vi "Get Codec - copy.vi"(8 "error in (no error)":errorcluster, 10 "Codec In":string, 11 "Absolute Path":path) -> (0 "error out":errorcluster, 3 "Codec Out":string)   [LabVIEW 2020]
doc: "Determines supported audio codec name based on file extension or wired in codec string."
uses:
  <vilib>/Utility/error.llb/Error Cluster From Error Code.vi
  <vilib>/ErrorRing/Error Ring.xnode
  <vilib>/Dataflow_G/G-Audio/G-Audio.lvlib
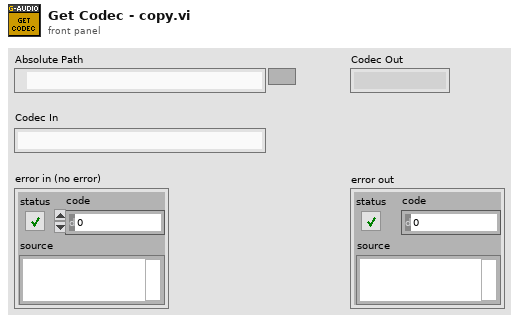
[diagram p1: front panel]
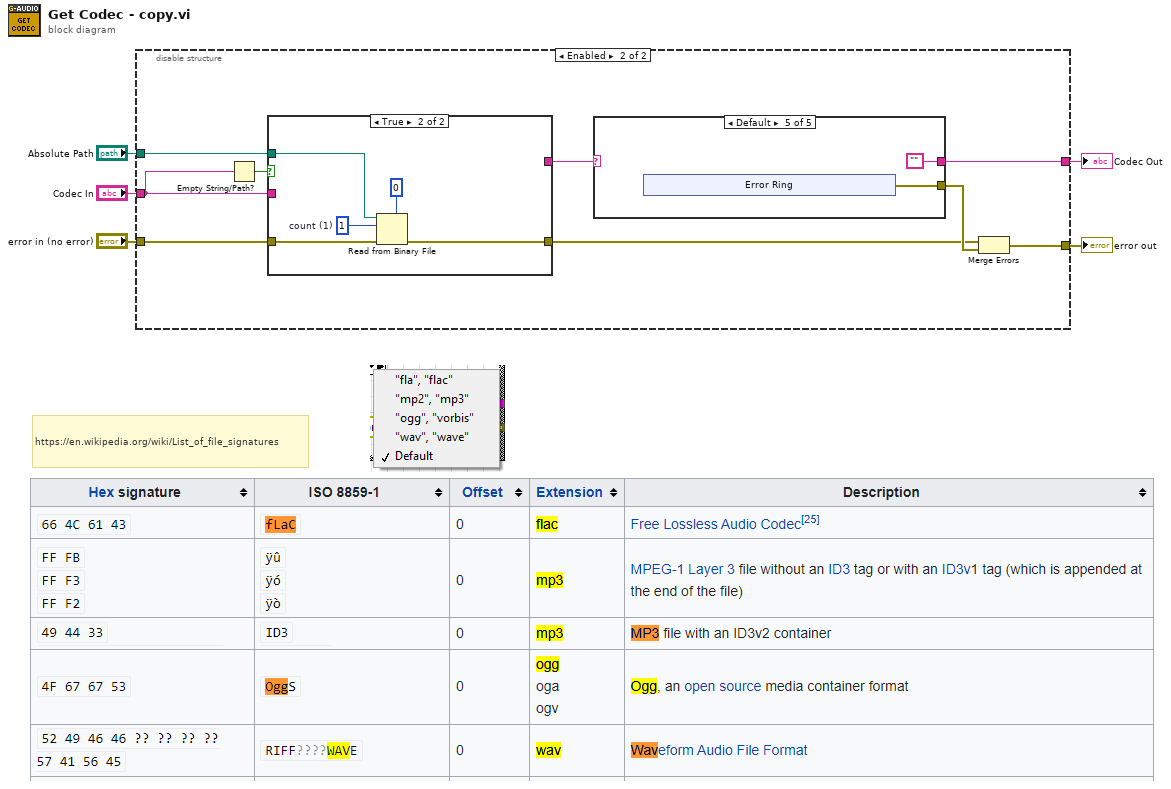
[diagram p0: block diagram]
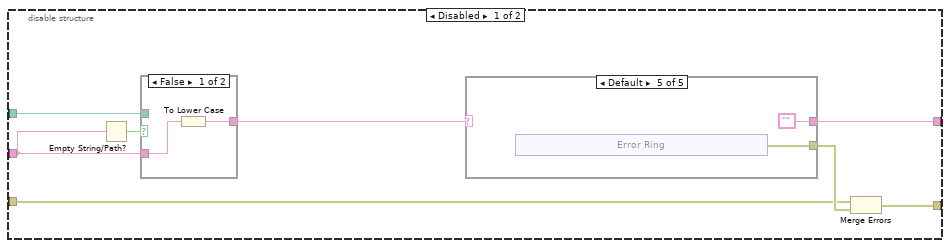
[diagram p2: hidden frame]
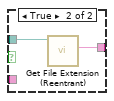
[diagram p3: hidden frame]
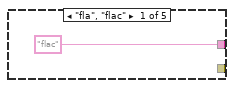
[diagram p4: hidden frame]
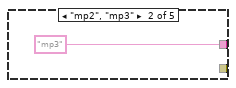
[diagram p5: hidden frame]
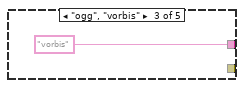
[diagram p6: hidden frame]
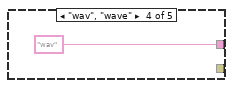
[diagram p7: hidden frame]
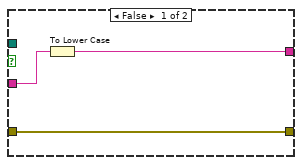
[diagram p8: hidden frame]
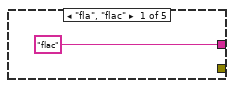
[diagram p9: hidden frame]
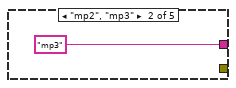
[diagram p10: hidden frame]
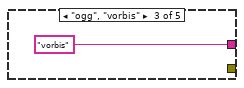
[diagram p11: hidden frame]
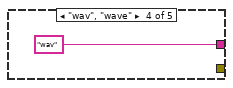
[diagram p12: hidden frame]
diagram:
  # "https://en.wikipedia.org/wiki/List_of_file_signatures"
  n1 = disable-structure shown="Enabled" {
    disable-tunnel: "Absolute Path" -> [w12 w36]
    disable-tunnel: "Codec In" -> [w10 w34]
    disable-tunnel: [w9 w33] -> w3
    disable-tunnel: "error in (no error)" -> [w7 w30]
    disable-tunnel: [w6 w31] -> w1
    frame Disabled {
      n2 = Empty String/Path?(string/path=w10) -> (empty?=w13:bool)
      n3 = case shown="False" w13 {
        tunnel: w12 -> [_ w17]
        tunnel: [w14 w16] -> w11
        tunnel: w10 -> [w15 _]
        frame False {
          n4 = To Lower Case(string=w15) -> (all lower case string=w14:string)
        }
        frame True {
          n5 = call <vilib>:"Get File Extension (Reentrant).vi"("file"=w17) -> ("lowercase file extension"=w16:string)  [unwired: 6 in, 4 out]
        }
      }
      n6 = case shown="Default" w11 {
        tunnel: ["flac" ("lowercase file extension") "mp3" ("lowercase file extension") "vorbis" ("lowercase file extension") "wav" ("lowercase file extension") "" ("lowercase file extension")] -> w9
        tunnel: [_ _ _ _ w22] -> w8
        frame "fla", "flac" {
        }
        frame "mp2", "mp3" {
        }
        frame "ogg", "vorbis" {
        }
        frame "wav", "wave" {
        }
        frame Default {
          n7 = xnode ("Error Ring")() -> ("error out"=w22:errorcluster)
        }
      }
      n8 = Merge Errors(w7, w8) -> (w6:errorcluster)
    }
    frame Enabled {
      n9 = Empty String/Path?(string/path=w34) -> (empty?=w37:bool)
      n10 = case shown="True" w37 {
        tunnel: w36 -> [_ w44]
        tunnel: [w39 _] -> w35
        tunnel: w34 -> [w40 _]
        tunnel: w30 -> [w38 w45]
        tunnel: [w38 w43] -> w29
        frame False {
          n11 = To Lower Case(string=w40) -> (all lower case string=w39:string)
        }
        frame True {
          w41 = 1  # count (1)
          n12 = Read from Binary File(5:u8 0, 8:w45, 10:w41, 11:w44) -> (0:w43:errorcluster)  [unwired: 2 in, 3 out]
        }
      }
      n13 = case shown="Default" w35 {
        tunnel: ["flac" ("lowercase file extension") "mp3" ("lowercase file extension") "vorbis" ("lowercase file extension") "wav" ("lowercase file extension") "" ("lowercase file extension")] -> w33
        tunnel: [_ _ _ _ w50] -> w32
        frame "fla", "flac" {
        }
        frame "mp2", "mp3" {
        }
        frame "ogg", "vorbis" {
        }
        frame "wav", "wave" {
        }
        frame Default {
          n14 = xnode ("Error Ring")() -> ("error out"=w50:errorcluster)
        }
      }
      n15 = Merge Errors(w29, w32) -> (w31:errorcluster)
    }
  }
  "Codec Out" <- w3
  "error out" <- w1
